vi "Read System State.vi"(8 "error in (no error)":errorcluster, 11 "System Actor in":refnum<class "System Actor.lvclass">) -> (0 "error out":errorcluster, 2 "System Status":T1 {"Command Processor Status"."Commands Behind" scale=0.0..10.0; "Command Processor Status"."Queued Commands" scale=0.0..100.0}, 3 "System Actor out":refnum<class "System Actor.lvclass">)   [LabVIEW 2014, in "Robot Actor Framework.lvlib" / "System Actor.lvlib" / "System Actor.lvclass"]
uses:
  System Actor.lvclass
  System State.ctl
  Command Actor/Command Actor Class/Command State.ctl
  Command Actor/Command Actor Class/Command States.ctl
  Command Processor Actor/Command Processor Actor Class/Command Processor State.ctl
  Command Processor Actor/Command Processor Actor Class/Command Processor States.ctl
  System Actor.lvclass/System Actor.ctl
  Command Actor/Command Actor Class/Command Actor.lvclass
  Command Processor Actor/Command Processor Actor Class/Command Processor Actor.lvclass
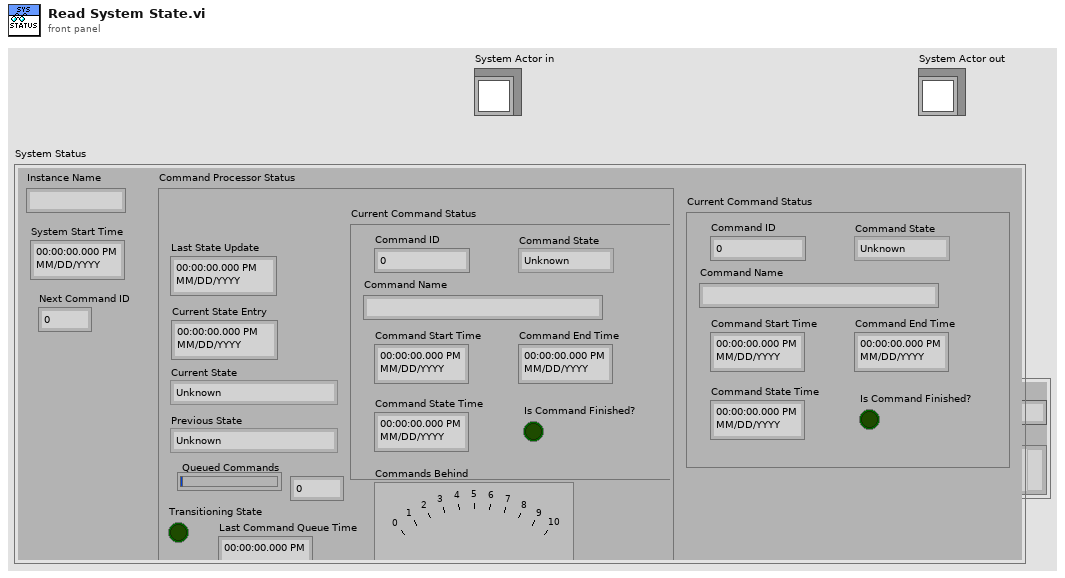
[diagram p1: front panel]
types:
  T1 = typedef "Robot Actor Framework.lvlib/System Actor.lvlib/System Actor.lvclass/System State.ctl" = cluster{"Instance Name":string, "Current Command Status":T2, "System Start Time":timestamp, "Next Command ID":dbl, "Command Processor Status":T4}
  T2 = typedef "Robot Actor Framework.lvlib/Command Actor.lvlib/Command Actor.lvclass/Command State.ctl" = cluster{"Command Name":string, "Command Start Time":timestamp, "Command End Time":timestamp, "Is Command Finished?":bool, "Command ID":u32, "Command State":T3, "Command State Time":timestamp}
  T3 = typedef "Robot Actor Framework.lvlib/Command Actor.lvlib/Command Actor.lvclass/Command States.ctl" = enum16{"Unknown", "Started", "Stopped", "Finished"}
  T4 = typedef "Robot Actor Framework.lvlib/Command Processor Actor.lvlib/Command Processor Actor.lvclass/Command Processor State.ctl" = cluster{"Current State":T5, "Last State Update":timestamp, "Queued Commands":u32, "Current Command Status":T2, "Previous State":T5, "Current State Entry":timestamp, "Transitioning State":bool, "Commands Behind":dbl, "Last Command Queue Time":timestamp}
  T5 = typedef "Robot Actor Framework.lvlib/Command Processor Actor.lvlib/Command Processor Actor.lvclass/Command Processor States.ctl" = enum16{"Unknown", "No Command", "Running Command", "Starting Command", "Stopping Command", "Finishing Command"}
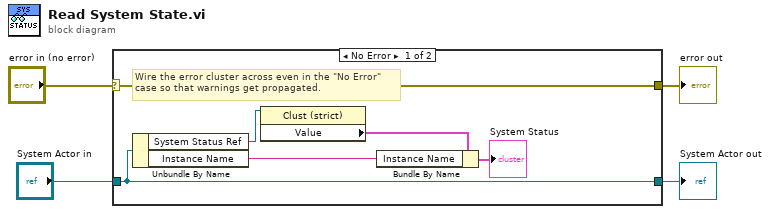
[diagram p0: block diagram]
diagram:
  n1 = case shown="No Error" "error in (no error)" {
    selector: "error in (no error)" -> [w10 w12]
    tunnel: [w10 w12] -> w3
    tunnel: [w9 w11] -> w1
    tunnel: "System Actor in" -> [w9 w11]
    frame No Error {
      # "Wire the error cluster across even in the \"No Error\"\ncase so that warnings get propagated."
      n2 = Unbundle By Name(w9) -> ("System Status Ref"=w8:refnum<vi>, "Instance Name"=w5:string)
      n3 = property class="Clust (strict)"(reference=w8) -> ("Value"=w7:T1)  [unwired: 1 in, 2 out]
      n4 = Bundle By Name(cluster=w7, "Instance Name"=w5) -> (→"System Status":T1)
    }
    frame Error {
    }
  }
  "error out" <- w3
  "System Actor out" <- w1
